vi "DATABASE.vi"(4 "error in (no error)":errorcluster, 5 "saving":bool, 6 "connection reference":T1, 7 "mask led":bool=TRUE) -> (0 "error out":errorcluster, 2 "connection reference out":T1)   [LabVIEW 2020]
doc: "This VI uses Data Base Connectivity Tools to connect with database hosted on a server using .udl flie. The current date is stored to the data base every 5 seconds after mask led boolean input is set to true."
uses:
  <vilib>/addons/database/Connection.llb/Conn ObjectReference.ctl
  <vilib>/addons/database/NI_Database_API.lvlib
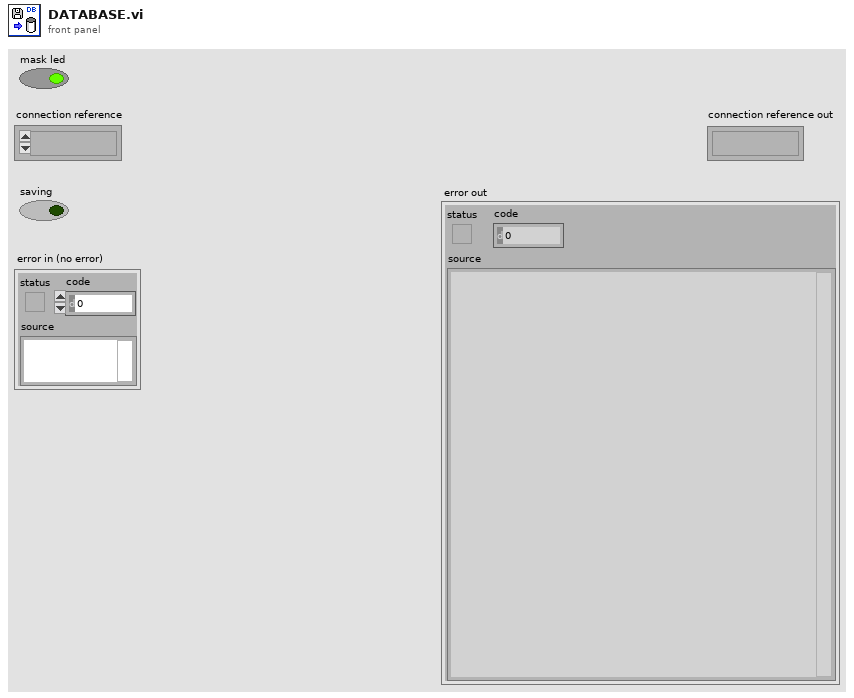
[diagram p1: front panel]
types:
  T1 = typedef "NI_Database_API.lvlib/Conn ObjectReference.ctl" = refnum<k1>
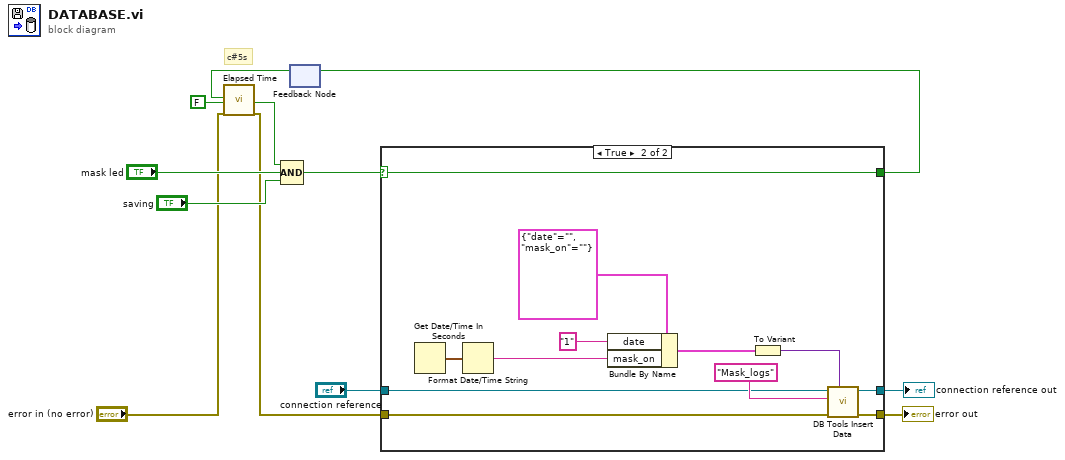
[diagram p0: block diagram]
diagram:
  # "c#5s"
  n1 = feedback #1() -> (w9:bool)  [unwired: 1 in]
  n2 = call "Elapsed Time"("Reset"=w9, "Auto Reset"=FALSE, "error in (no error)"="error in (no error)") -> ("Time has Elapsed"=w5:bool, "error out"=w1:errorcluster)  [unwired: 9 in, 6 out]
  n3 = Compound Arithmetic op=AND(w5, "mask led", "saving") -> (w6:bool)
  n4 = case shown="True" w6 {
    selector: w6 -> [_ w17]
    tunnel: "connection reference" -> [w14 w19]
    tunnel: [w14 w18] -> w11
    tunnel: [_ w17] -> w8
    tunnel: w1 -> [w13 w16]
    tunnel: [w13 w15] -> w7
    frame False {
    }
    frame True {
      n5 = Get Date/Time In Seconds() -> (seconds since 1Jan1904=w24:timestamp)
      n6 = Format Date/Time String(seconds (now)=w24) -> (date/time string=w20:string)  [unwired: 2 in]
      n7 = Bundle By Name(cluster=cluster{"date":string, "mask_on":string} {"date"="", "mask_on"=""}, "date"="1" ("mask_on"), "mask_on"=w20) -> (w23:cluster{"date":string, "mask_on":string})
      n8 = To Variant(anything=w23) -> (Variant=w22:variant)
      n9 = call <vilib>:"DB Tools Insert Data.vi"("data"=w22, "error in (no error)"=w16, "table"="Mask_logs", "connection reference"=w19) -> ("error out"=w15:errorcluster, "connection reference out"=w18:T1)  [unwired: 6 in]
    }
  }
  "connection reference out" <- w11
  "error out" <- w7
  n10 = feedback-in #1(w8) -> ()
